vi "Read.vi"(8 "error in (no error)":errorcluster, 11 "Const_Variant in":refnum<class "Const_Variant.lvclass">) -> (0 "error out":errorcluster, 2 "Variant":variant, 3 "Const_Variant out":refnum<class "Const_Variant.lvclass">)   [LabVIEW 2021, in "Const_Variant.lvclass"]
uses:
  Const_Variant.lvclass
  Const_Variant.lvclass/Const_Variant.ctl
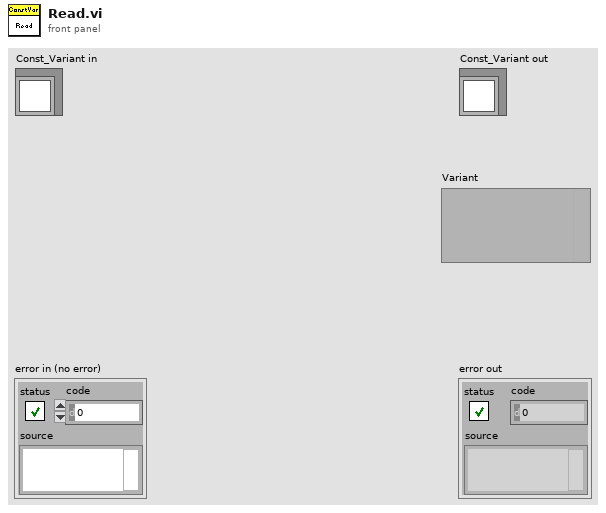
[diagram p1: front panel]
types:
  T1 = typedef "Const_Variant.lvclass/Type.ctl" = variant
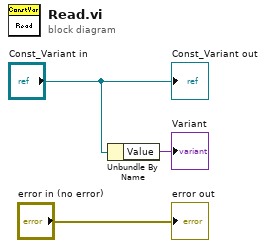
[diagram p0: block diagram]
diagram:
  n1 = Unbundle By Name("Const_Variant in") -> ("Value"=→"Variant":T1)
  "error out" <- "error in (no error)"
  "Const_Variant out" <- "Const_Variant in"
